vi "用户登录查询.vi"(10 "密码":string, 11 "用户名":string) -> (0 "error out":errorcluster, 3 "text":string)   [LabVIEW 2014]
uses:
  <vilib>/httpClient/MultipartData.ctl
  <vilib>/httpClient/LabVIEWHTTPClient.lvlib
panel:
  out "ServerResponseBody_UTF8":string
  out "ServerResponseHead":string
  out "resulting string":string
  out "ServerResponseBody_ANSI":string
  out "上传成功":bool
  out "添加的路径":path
  in  "error in (no error)":errorcluster caption="错误输入（无错误）"
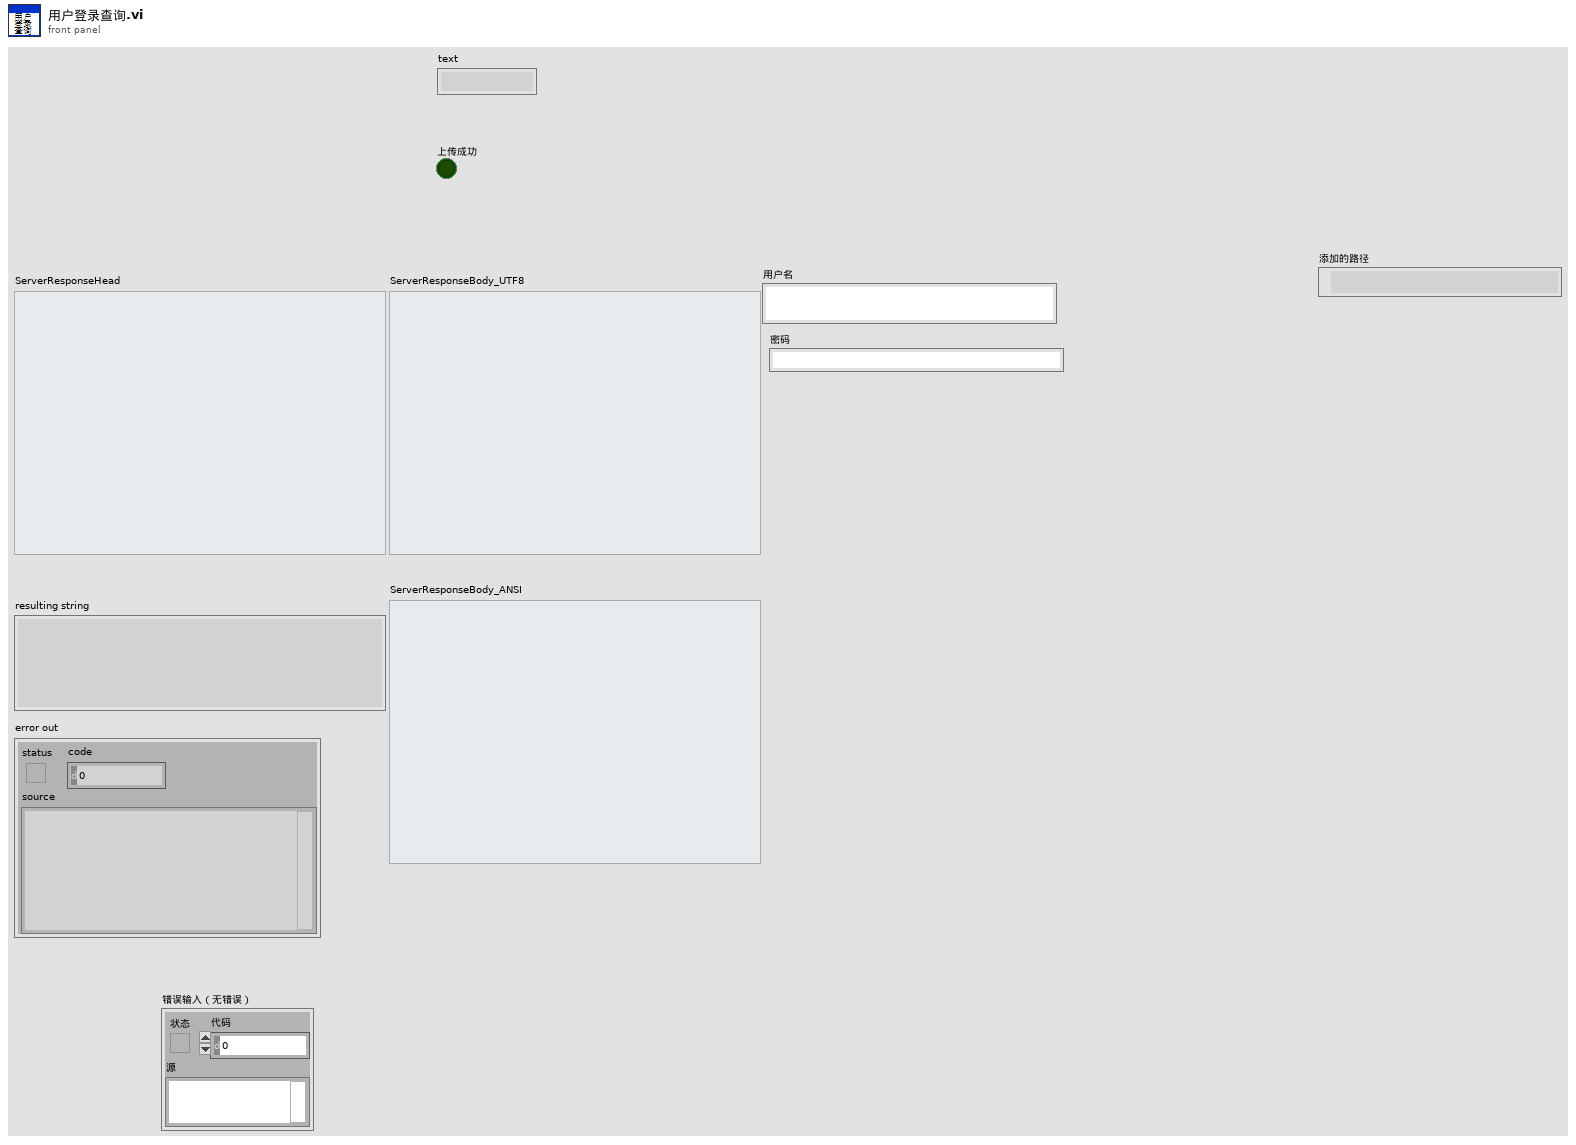
[diagram p1: front panel]
types:
  T1 = typedef "LabVIEWHTTPClient.lvlib/MultipartData.ctl" = cluster{"Name":string, "Value":string, "File":path, "Filename":string, "MIME type":string}
  T2 = typedef "LabVIEWHTTPClient.lvlib/ClientHandle.ctl" = refnum<k1>
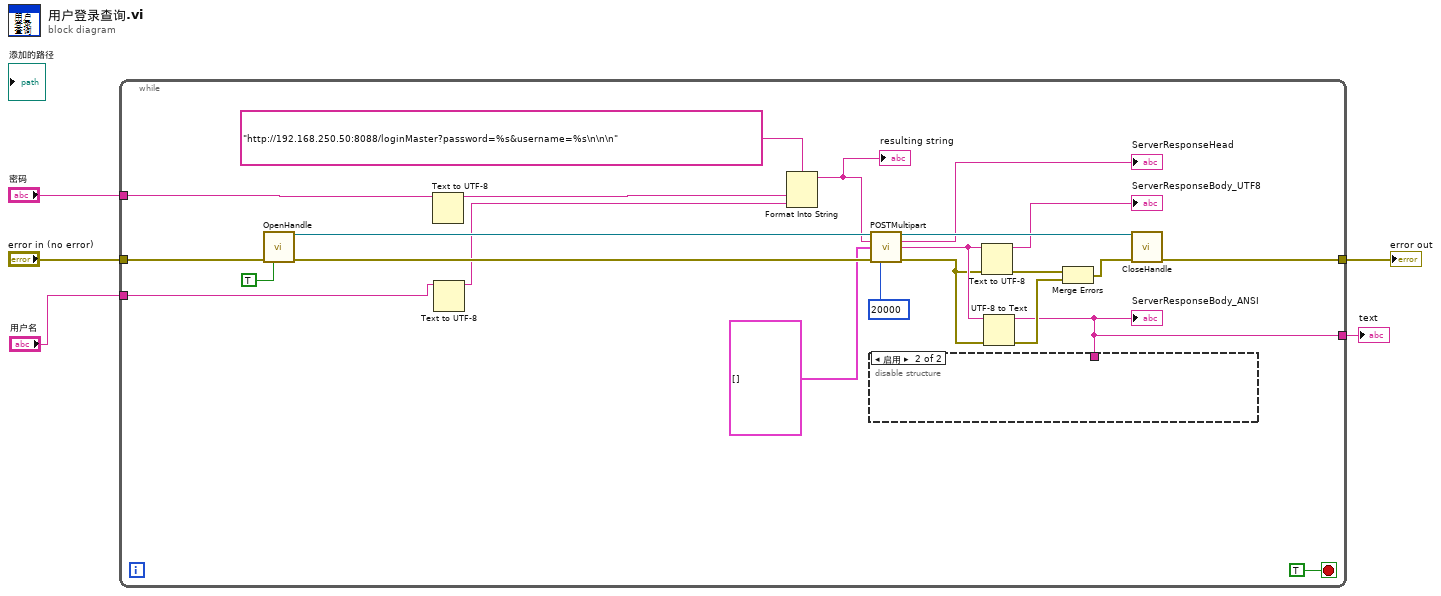
[diagram p0: block diagram]
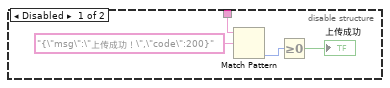
[diagram p2: hidden frame]
diagram:
  n1 = while {
    tunnel: "密码" -> [w11]
    tunnel: "用户名" -> [w7]
    tunnel: [w6] -> w1
    tunnel: "error in (no error)" -> [w16]
    tunnel: [w18] -> w5
    stop <- TRUE stop-if-true
    n2 = call <vilib>:"OpenHandle.vi"("error in (no error)"=w16, "verify server(true)"=TRUE) -> ("client handle out"=w13:T2, "error out"=w28:errorcluster)  [unwired: 12 in]
    n3 = Text to UTF-8(11:w11) -> (3:w10:string)  [unwired: 2 in, 1 out]
    n4 = Text to UTF-8(11:w7) -> (3:w8:string)  [unwired: 2 in, 1 out]
    n5 = Format Into String(format string="http://192.168.250.50:8088/loginMaster?password=%s&username=%s\n\n\n" ("url"), w10, w8) -> (resulting string=w9:string)  [unwired: 2 in, 1 out]
    "resulting string" <- w9
    n6 = call <vilib>:"POSTMultipart.vi"("client handle"=w13, "url"=w9, "data"=T1[] [], "error in (no error)"=w28, "timeout (10000)"=20000) -> ("client handle out"=w27:T2, "headers"=→"ServerResponseHead":string, "body"=w22:string, "error out"=w21:errorcluster)  [unwired: 7 in]
    n7 = Text to UTF-8(8:w21, 11:w22) -> (0:w20:errorcluster, 3:→"ServerResponseBody_UTF8":string)  [unwired: 1 in]
    n8 = UTF-8 to Text(8:w21, 11:w22) -> (0:w17:errorcluster, 3:w6:string)  [unwired: 1 in]
    "ServerResponseBody_ANSI" <- w6
    n9 = disable-structure shown="启用" {
      disable-tunnel: w6 -> [w29 _]
      frame Disabled {
        n10 = Match Pattern(string=w29, regular expression="{\"msg\":\"上传成功！\",\"code\":200}" ("正则表达式")) -> (offset past match=w31:i32)  [unwired: 1 in, 3 out]
        n11 = Greater Or Equal To 0?(x=w31) -> (x >= 0?=→"上传成功":bool)
      }
      frame Enabled {
      }
    }
    n12 = Merge Errors(w20, w17) -> (w19:errorcluster)
    n13 = call <vilib>:"CloseHandle.vi"("client handle"=w27, "error in (no error)"=w19) -> ("error out"=w18:errorcluster)  [unwired: 13 in]
  }
  "error out" <- w5
  "text" <- w1
